vi "Perform Action.vi"(8 "error in":errorcluster, 10 "Input":variant, 11 "AO DAQmx DC CFG in":refnum<class "AO DAQmx DC CFG.lvclass">) -> (0 "error out":errorcluster, 2 "Output":variant, 3 "AO DAQmx DC CFG out":refnum<class "AO DAQmx DC CFG.lvclass">)   [LabVIEW 2024, in "AO DAQmx DC CFG.lvclass"]
uses:
  AO DAQmx DC CFG.lvclass
  DAQmx Base CFG/DAQmx Base CFG.lvclass/DAQmx Base CFG.ctl
  AO DAQmx DC CFG.lvclass/AO DAQmx DC CFG.ctl
  <vilib>/DAQmx/miscellaneous.llb/DAQmx Fill In Error Info.vi
  <vilib>/DAQmx/write.llb/DAQmx Write (Analog 1D DBL NChan 1Samp).vi
  Buffers/BufferWrites1SamDBL/BufferWrites1SamDBL.lvclass
  DAQmx Base CFG/DAQmx Base CFG.lvclass
  D:/git/HAL/HAL/Devices/DAQmx/DAQmx Base CFG/DAQmx Base CFG.lvclass
  D:/git/HAL/HAL/Configurations/CFG JSON/CFG JSON.lvclass
  D:/git/HAL/HAL/Configurations/CFG Base/CFG Base.lvclass
  D:/git/HAL/HAL/Devices/DAQmx/AO/AO DAQmx DC CFG/AO DAQmx DC CFG.lvclass
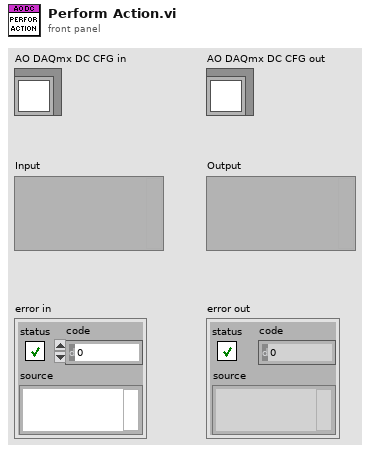
[diagram p1: front panel]
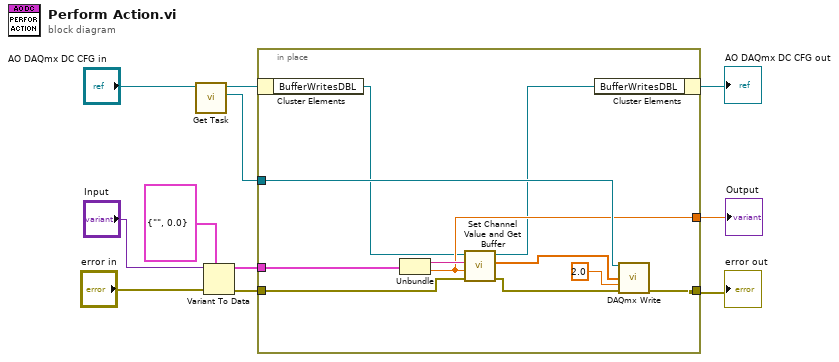
[diagram p0: block diagram]
diagram:
  n1 = call "Get Task.vi"("DAQmx Base CFG in"="AO DAQmx DC CFG in") -> ("Task"=w4:refnum<k21>, "DAQmx Base CFG out"=w2:refnum<class "AO DAQmx DC CFG.lvclass">)  [unwired: 9 in]
  n2 = Variant To Data(error in="error in", type=cluster{"Channel":string, "Level":dbl} {"Channel"="", "Level"=0.0}, Variant="Input") -> (data=w7:cluster{"Channel":string, "Level":dbl}, error out=w8:errorcluster)
  n3 = in-place {
    in-place-border: w8 -> [w15]
    in-place-border: w7 -> [w22]
    in-place-border: [w20] -> w5
    in-place-border: w4 -> [w19]
    in-place-border: [w16] -> w3
    n4 = in-place-cluster #1(w2) -> ("BufferWritesDBL"=w14:refnum<class "BufferWrites1SamDBL.lvclass">)
    n5 = Unbundle(w22) -> ("Channel"=w18:string, "Level"=w16:dbl)
    n6 = call-dynamic "Set Channel Value and Get Buffer.vi"("error in"=w15, "Value"=w16, "Channel"=w18, "BufferWritesDBL in"=w14) -> ("error out"=w12:errorcluster, "Write Buffer"=w21:dbl[], "BufferWritesDBL out"=w13:refnum<class "BufferWrites1SamDBL.lvclass">)  [unwired: 5 in]
    n7 = in-place-cluster #1("BufferWritesDBL"=w13) -> (→"AO DAQmx DC CFG out":refnum<class "AO DAQmx DC CFG.lvclass">)
    n8 = call-poly <vilib>:"DAQmx Write.vi"("task/channels in"=w19, "data"=w21, "timeout"=2.0, "error in"=w12) -> ("error out"=w20:errorcluster)  [unwired: 9 in, 2 out]
  }
  "error out" <- w5
  "Output" <- w3
